vi "Test DUT Self Test Without Wait for Reply Does not Cause Error.vi"(8 "error in (no error)":errorcluster, 11 "Device Under Test Test In":refnum<class "Device Under Test Test.lvclass">) -> (0 "error out":errorcluster, 3 "Device Under Test Test Out":refnum<class "Device Under Test Test.lvclass">)   [LabVIEW 2020, in "Device Under Test Test.lvclass"]
uses:
  Device Under Test Test.lvclass
  Device Under Test/Device Under Test.lvclass
  <vilib>/Asteme/Triarc Framework/Process/Process.lvclass
  C:/Program Files (x86)/National Instruments/LabVIEW 2020/vi.lib/Asteme/Triarc Framework/View/View.lvclass
  C:/Program Files (x86)/National Instruments/LabVIEW 2020/vi.lib/Asteme/Triarc Framework/Process/Process.lvclass
  C:/Program Files (x86)/National Instruments/LabVIEW 2020/vi.lib/Asteme/Triarc Framework/Base/Base.lvclass
  C:/Program Files (x86)/National Instruments/LabVIEW 2020/vi.lib/Asteme/Triarc Framework/Error Handler Interface/Error Handler Interface.lvclass
  C:/Program Files (x86)/National Instruments/LabVIEW 2020/vi.lib/Asteme/Triarc Framework/Logging/Logging.lvclass
  C:/Users/anton/Documents/GitHub/Triarc-Examples/Thermal Chamber/Device Under Test/Device Under Test.lvclass
  <vilib>/Asteme/Triarc Framework Test Suite/Mock Error Handler/Mock Error Handler.lvclass
  <vilib>/Asteme/LUnit/Test Case.lvclass
  C:/Program Files (x86)/National Instruments/LabVIEW 2020/vi.lib/Asteme/Triarc Framework Test Suite/Mock Error Handler/Mock Error Handler.lvclass
  C:/Program Files (x86)/National Instruments/LabVIEW 2020/vi.lib/Asteme/Triarc Framework Test Suite/View Test/View Test.lvclass
  C:/Program Files (x86)/National Instruments/LabVIEW 2020/vi.lib/Asteme/Triarc Framework Test Suite/Process Test/Process Test.lvclass
  C:/Program Files (x86)/National Instruments/LabVIEW 2020/vi.lib/Asteme/Triarc Framework Test Suite/Base Class Test/Base Test.lvclass
  C:/Program Files (x86)/National Instruments/LabVIEW 2020/vi.lib/Asteme/LUnit/Test Case.lvclass
  C:/Users/anton/Documents/GitHub/Triarc-Examples/Thermal Chamber/Device Under Test Test/Device Under Test Test.lvclass
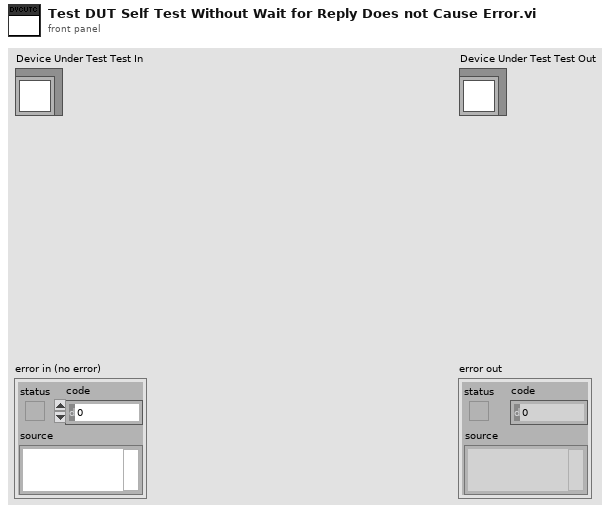
[diagram p1: front panel]
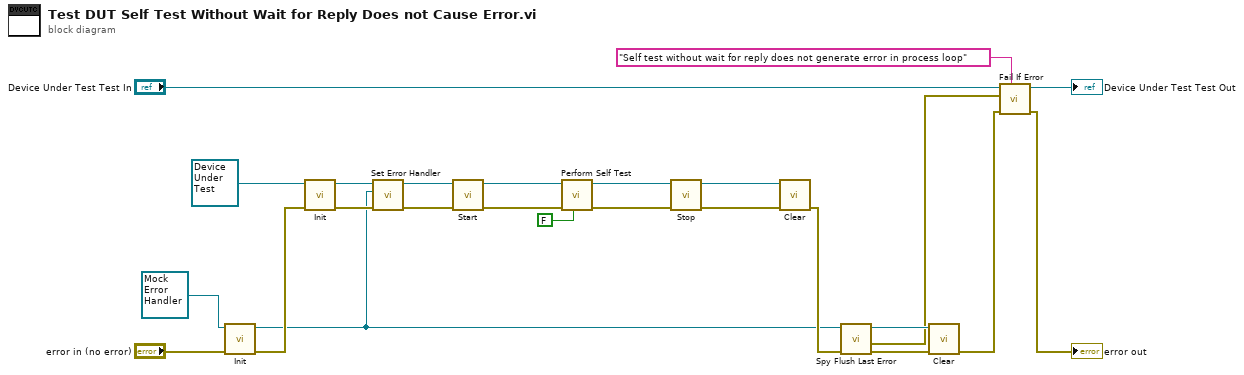
[diagram p0: block diagram]
diagram:
  n1 = call-dynamic "Init.vi"("error in (no error)"="error in (no error)", "Mock Error Handler In"=refnum<class "Mock Error Handler.lvclass"> refnum ("TFTS.lvlib:Mock Error Handler.lvclass")) -> ("error out"=w11:errorcluster, "Mock Error Handler Out"=w8:refnum<class "Mock Error Handler.lvclass">)  [unwired: 8 in]
  n2 = call-dynamic "Init.vi"("error in (no error)"=w11, "View In"=refnum<class "Device Under Test.lvclass"> refnum ("Device Under Test.lvclass")) -> ("error out"=w14:errorcluster, "View Out"=w16:refnum<class "Device Under Test.lvclass">)  [unwired: 8 in]
  n3 = call <vilib>:"Set Error Handler.vi"("error in (no error)"=w14, "Error Handler"=w8, "Process In"=w16) -> ("error out"=w13:errorcluster, "Process Out"=w15:refnum<class "Device Under Test.lvclass">)  [unwired: 7 in]
  n4 = call <vilib>:"Start.vi"("error in (no error)"=w13, "Process In"=w15) -> ("error out"=w23:errorcluster, "Process Out"=w24:refnum<class "Device Under Test.lvclass">)  [unwired: 8 in]
  n5 = call "Perform Self Test.vi"("Wait for Reply?"=FALSE, "error in (no error)"=w23, "Device Under Test In"=w24) -> ("error out"=w21:errorcluster, "Device Under Test Out"=w22:refnum<class "Device Under Test.lvclass">)  [unwired: 5 in, 2 out]
  n6 = call <vilib>:"Stop.vi"("error in (no error)"=w21, "Process In"=w22) -> ("error out"=w19:errorcluster, "Process Out"=w20:refnum<class "Device Under Test.lvclass">)  [unwired: 7 in, 1 out]
  n7 = call-dynamic "Clear.vi"("error in (no error)"=w19, "View In"=w20) -> ("error out"=w10:errorcluster)  [unwired: 9 in]
  n8 = call <vilib>:"Spy Flush Last Error.vi"("error in (no error)"=w10, "Mock Error Handler In"=w8) -> ("error out"=w9:errorcluster, "Error"=w2:errorcluster, "Mock Error Handler Out"=w7:refnum<class "Mock Error Handler.lvclass">)  [unwired: 7 in]
  n9 = call-dynamic "Clear.vi"("error in (no error)"=w9, "Mock Process In"=w7) -> ("error out"=w3:errorcluster)  [unwired: 9 in]
  n10 = call <vilib>:"Fail If Error.vi"("Description"="Self test without wait for reply does not generate error in process loop", "error in (no error)"=w3, "Assert error"=w2, "Test Case In"="Device Under Test Test In") -> ("error out"=→"error out":errorcluster, "Test Case Out"=→"Device Under Test Test Out":refnum<class "Device Under Test Test.lvclass">)  [unwired: 6 in]
